vi "segurito.vi"(1 "start":dbl, 2 "change":dbl) -> (0 "output":dbl)   [LabVIEW 2020]
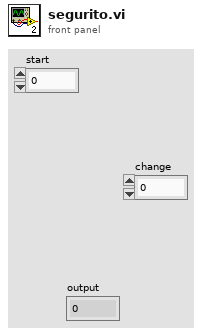
[diagram p1: front panel]
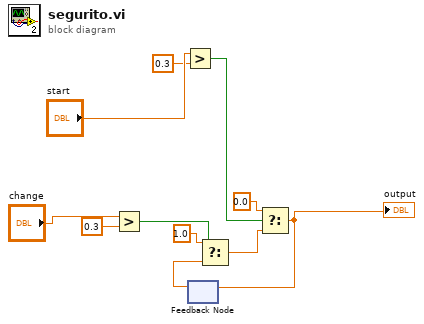
[diagram p0: block diagram]
diagram:
  n1 = Greater?(x="change", y=0.3) -> (0:w5:bool)
  n2 = Greater?(x="start", y=0.3) -> (0:w6:bool)
  n3 = feedback #1() -> (w10:dbl)  [unwired: 1 in]
  n4 = Select(t=1.0, s=w5, f=w10) -> (s? t:f=w7:dbl)
  n5 = Select(t=0.0, s=w6, f=w7) -> (s? t:f=w8:dbl)
  "output" <- w8
  n6 = feedback-in #1(w8) -> ()
